vi "Call Notifier.vi"(8 "error in (no error)":errorcluster, 10 "ID":i64=-9223372036854775808 format="%.0p", 11 "Map Notifier Controller in":refnum<class "Map Notifier Controller.lvclass">) -> (0 "error out":errorcluster, 1 "Key Not Found?":bool, 2 "Notifier Out":refnum<class "Notifier.lvclass">, 3 "Map Notifier Controller out":refnum<class "Map Notifier Controller.lvclass">)   [LabVIEW 2024, in "Map Notifier Controller.lvclass"]
uses:
  Map Notifier Controller.lvclass
  Ancestor Class/Actor Assistant/Notifier/Notifier.lvclass
  Map Notifier Controller.lvclass/Map Notifier Controller.ctl
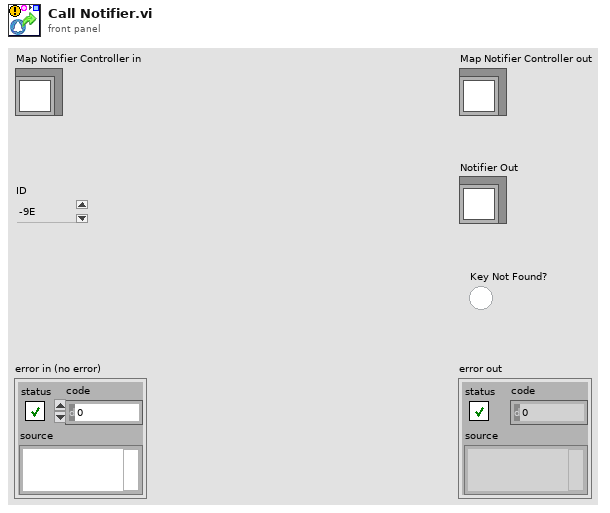
[diagram p1: front panel]
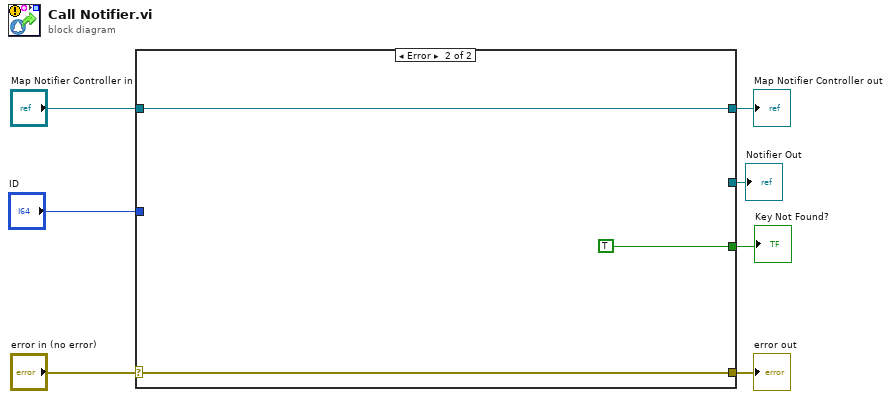
[diagram p0: block diagram]
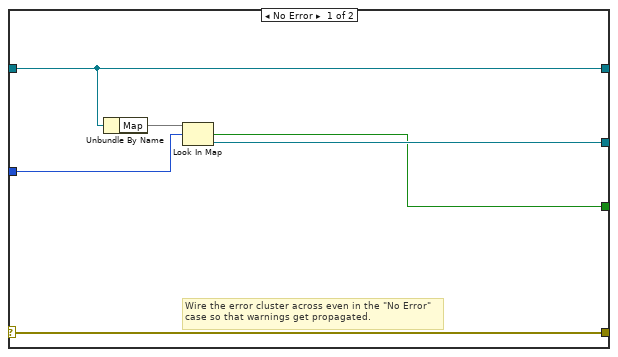
[diagram p2: hidden frame]
diagram:
  n1 = case shown="Error" "error in (no error)" {
    selector: "error in (no error)" -> [w13 w16]
    tunnel: [w13 w16] -> w6
    tunnel: [w12 w15] -> w4
    tunnel: "Map Notifier Controller in" -> [w12 w15]
    tunnel: "ID" -> [w10 _]
    tunnel: [w9 _] -> w2
    tunnel: [w8 TRUE ("key not found?")] -> w1
    frame No Error {
      # "Wire the error cluster across even in the \"No Error\"\ncase so that warnings get propagated."
      n2 = Unbundle By Name(w12) -> ("Map"=w11:map{i64, refnum<class "Notifier.lvclass">})
      n3 = Look In Map(map=w11, key=w10) -> (key not found?=w8:bool, value=w9:refnum<class "Notifier.lvclass">)  [unwired: 1 in]
    }
    frame Error {
    }
  }
  "error out" <- w6
  "Map Notifier Controller out" <- w4
  "Notifier Out" <- w2
  "Key Not Found?" <- w1
